vi "time-temp_to_string.vi"(0 "Time":timestamp, 3 "Temperature":dbl) -> (6 "String":string)   [LabVIEW 2017]
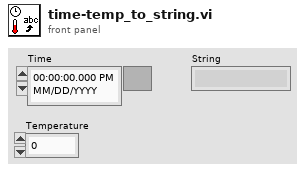
[diagram p1: front panel]
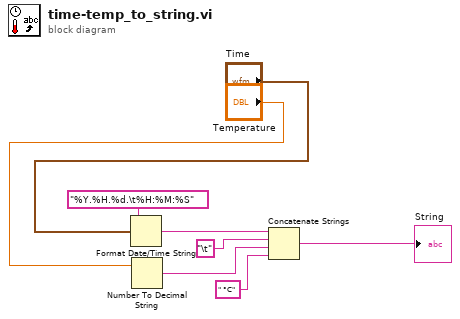
[diagram p0: block diagram]
diagram:
  n1 = Format Date/Time String(time format string (%c)="%Y.%H.%d.\t%H:%M:%S", seconds (now)="Time") -> (date/time string=w1:string)  [unwired: 1 in]
  n2 = Number To Decimal String(number="Temperature") -> (decimal integer string=w3:string)  [unwired: 1 in]
  n3 = Concatenate Strings(w1, "\t" ("string"), w3, " °C" ("string")) -> (→"String":string)
